vi "Divide Rectangle.vi"(7 "Band (50)":i16=50, 9 "Coords":T1={"Horizontal"=-10000, "Vertical"=-10000}, 11 "Rectangle":T2) -> (1 "Zone":i32=-1, 3 "Zones Rectangles":T3(array[cluster]))   [LabVIEW 2012]
doc: "Creates an array of nine \"Zones\" based on the Snap Band parameter (distance from boundaries).\n\nIf coordinates are supplied, the VI also calculates at which zone the coordinates are pointing. \n\n-1: outside of all zones\n0: center\n1: top-left\n2: top\n3: top-right\n4: left\n5: right\n6: bottom-left\n7: bottom\n8: bottom-right"
uses:
  <vilib>/Utility/miscctls.llb/LVPoint32TypeDef.ctl
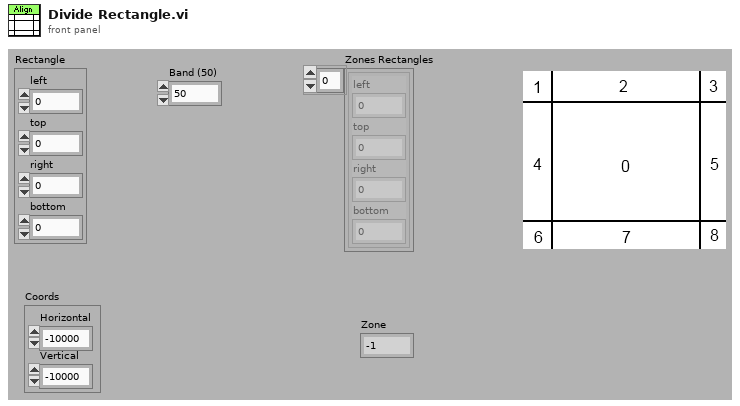
[diagram p1: front panel]
types:
  T1 = typedef "LVPoint32TypeDef.ctl" = cluster{"Horizontal":i32, "Vertical":i32}
  T2 = cluster{"left":i16, "top":i16, "right":i16, "bottom":i16}
  T3 = cluster{"left":i16, "top":i16, "right":i16, "bottom":i16}[]
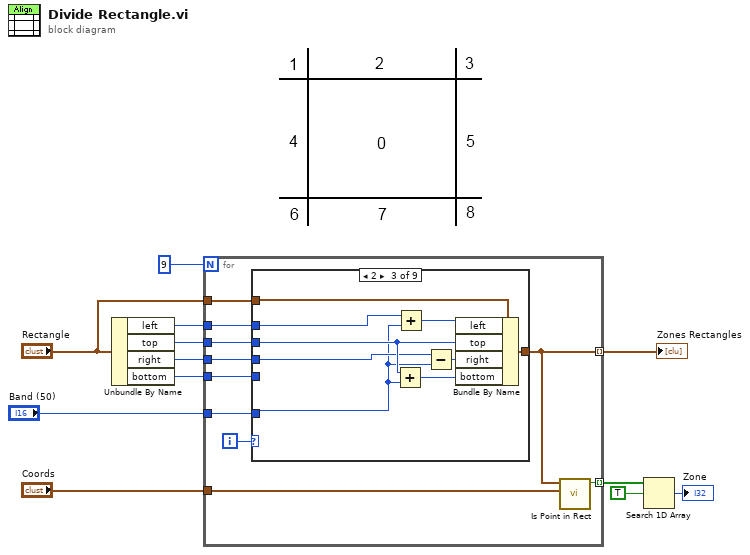
[diagram p0: block diagram]
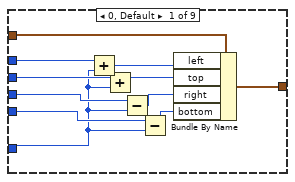
[diagram p2: hidden frame]
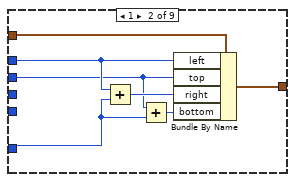
[diagram p3: hidden frame]
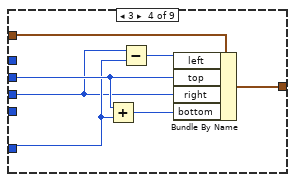
[diagram p4: hidden frame]
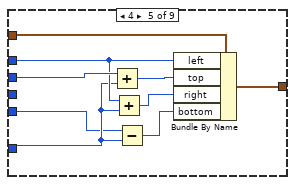
[diagram p5: hidden frame]
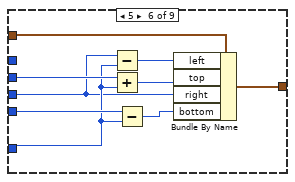
[diagram p6: hidden frame]
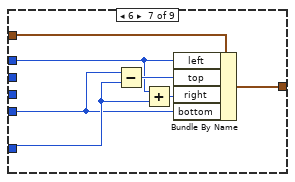
[diagram p7: hidden frame]
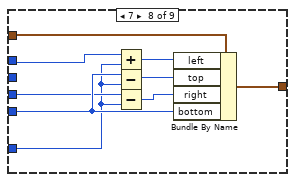
[diagram p8: hidden frame]
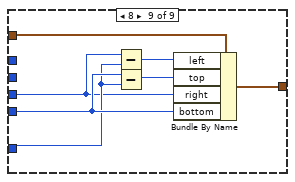
[diagram p9: hidden frame]
diagram:
  n1 = Unbundle By Name("Rectangle") -> ("left"=w6:i16, "top"=w7:i16, "right"=w8:i16, "bottom"=w9:i16)
  n2 = for {
    N: 9 -> [_]
    tunnel: w6 -> [w21]
    tunnel: w7 -> [w20]
    tunnel: w8 -> [w19]
    tunnel: w9 -> [w18]
    tunnel: "Rectangle" -> [w17]
    tunnel: "Band (50)" -> [w16]
    tunnel: [w15] -> w12 mode=indexing
    tunnel: "Coords" -> [w14]
    tunnel: [w13] -> w3 mode=indexing
    i -> [w22]
    n3 = case shown="2" w22 {
      tunnel: w21 -> [w31 w38 w47 _ w61 _ w78 w82 _]
      tunnel: w20 -> [w30 w36 w46 w54 w63 w72 _ _ _]
      tunnel: w19 -> [w27 _ w42 w50 _ w66 _ w85 w91]
      tunnel: w18 -> [w26 _ _ _ w58 w70 w75 w87 w94]
      tunnel: w17 -> [w33 w40 w49 w56 w65 w74 w81 w90 w97]
      tunnel: w16 -> [w25 w35 w41 w52 w60 w68 w77 w84 w92]
      tunnel: [w32 w39 w48 w55 w64 w73 w80 w89 w96] -> w15
      frame 0, Default {
        n4 = Add(x=w31, y=w25) -> (x+y=w29:i16)
        n5 = Add(x=w30, y=w25) -> (x+y=w28:i16)
        n6 = Subtract(x=w27, y=w25) -> (x-y=w24:i16)
        n7 = Subtract(x=w26, y=w25) -> (x-y=w23:i16)
        n8 = Bundle By Name(cluster=w33, "left"=w29, "top"=w28, "right"=w24, "bottom"=w23) -> (w32:T2)
      }
      frame 1 {
        n9 = Add(x=w38, y=w35) -> (x+y=w37:i16)
        n10 = Add(x=w36, y=w35) -> (x+y=w34:i16)
        n11 = Bundle By Name(cluster=w40, "left"=w38, "top"=w36, "right"=w37, "bottom"=w34) -> (w39:T2)
      }
      frame 2 {
        n12 = Add(x=w46, y=w41) -> (x+y=w45:i16)
        n13 = Add(x=w47, y=w41) -> (x+y=w44:i16)
        n14 = Subtract(x=w42, y=w41) -> (x-y=w43:i16)
        n15 = Bundle By Name(cluster=w49, "left"=w44, "top"=w46, "right"=w43, "bottom"=w45) -> (w48:T2)
      }
      frame 3 {
        n16 = Add(x=w54, y=w52) -> (x+y=w53:i16)
        n17 = Subtract(x=w50, y=w52) -> (x-y=w51:i16)
        n18 = Bundle By Name(cluster=w56, "left"=w51, "top"=w54, "right"=w50, "bottom"=w53) -> (w55:T2)
      }
      frame 4 {
        n19 = Add(x=w63, y=w60) -> (x+y=w62:i16)
        n20 = Add(x=w61, y=w60) -> (x+y=w59:i16)
        n21 = Subtract(x=w58, y=w60) -> (x-y=w57:i16)
        n22 = Bundle By Name(cluster=w65, "left"=w61, "top"=w62, "right"=w59, "bottom"=w57) -> (w64:T2)
      }
      frame 5 {
        n23 = Subtract(x=w66, y=w68) -> (x-y=w67:i16)
        n24 = Add(x=w72, y=w68) -> (x+y=w71:i16)
        n25 = Subtract(x=w70, y=w68) -> (x-y=w69:i16)
        n26 = Bundle By Name(cluster=w74, "left"=w67, "top"=w71, "right"=w66, "bottom"=w69) -> (w73:T2)
      }
      frame 6 {
        n27 = Subtract(x=w75, y=w77) -> (x-y=w79:i16)
        n28 = Add(x=w78, y=w77) -> (x+y=w76:i16)
        n29 = Bundle By Name(cluster=w81, "left"=w78, "top"=w79, "right"=w76, "bottom"=w75) -> (w80:T2)
      }
      frame 7 {
        n30 = Add(x=w82, y=w84) -> (x+y=w88:i16)
        n31 = Subtract(x=w87, y=w84) -> (x-y=w86:i16)
        n32 = Subtract(x=w85, y=w84) -> (x-y=w83:i16)
        n33 = Bundle By Name(cluster=w90, "left"=w88, "top"=w86, "right"=w83, "bottom"=w87) -> (w89:T2)
      }
      frame 8 {
        n34 = Subtract(x=w91, y=w92) -> (x-y=w95:i16)
        n35 = Subtract(x=w94, y=w92) -> (x-y=w93:i16)
        n36 = Bundle By Name(cluster=w97, "left"=w95, "top"=w93, "right"=w91, "bottom"=w94) -> (w96:T2)
      }
    }
    n37 = call "Is Point in Rect.vi"("point"=w14, "rect"=w15) -> ("Point in Rect?"=w13:bool)  [unwired: 9 out]
  }
  "Zones Rectangles" <- w12
  n38 = Search 1D Array(1D array=w3, element=TRUE) -> (index of element=→"Zone":i32)  [unwired: 1 out]
